vi "Setup Telem APIs.vi"(8 "error in (no error)":errorcluster, 11 "Volatus Core in":refnum<class "Volatus Core.lvclass">) -> (0 "error out":errorcluster, 3 "Volatus Core out":refnum<class "Volatus Core.lvclass">)   [LabVIEW 2020, in "Volatus.lvlib" / "Volatus Core.lvclass"]
uses:
  Volatus Core.lvclass
  C:/dev/lv20CE/relink/lv-volatus/Volatus/Module/Module.lvclass
  Volatus Core.lvclass/Volatus Core.ctl
  Module/Module.lvclass/Module.ctl
  VolatusAPI/VolatusAPI.lvclass/VolatusAPI.ctl
  Module/Module.lvclass
  lv-vecto/Vecto/Vecto/Vecto.lvclass
  VolatusAPI/VolatusAPI.lvclass
  C:/dev/lv20CE/relink/lv-volatus/Volatus/Volatus Core/Volatus Core.lvclass
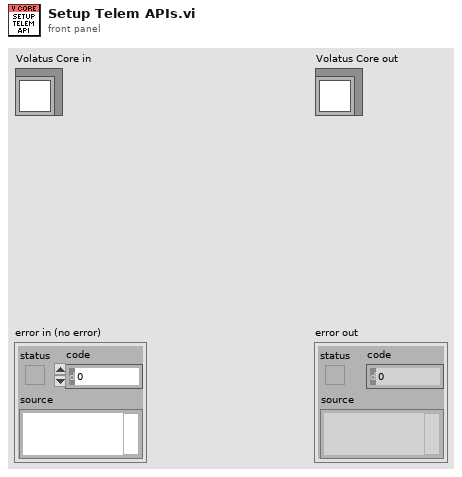
[diagram p1: front panel]
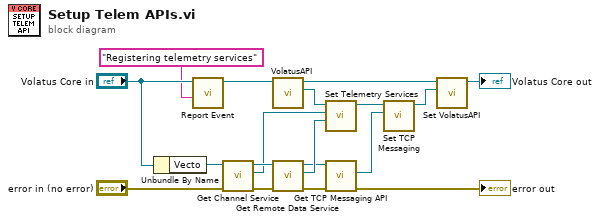
[diagram p0: block diagram]
diagram:
  n1 = Unbundle By Name("Volatus Core in") -> ("Vecto"=w16:refnum<class "Vecto.lvclass">)
  n2 = call "Report Event.vi"("Message"="Registering telemetry services", "Module in"="Volatus Core in") -> ("Module out"=w7:refnum<class "Volatus Core.lvclass">)  [unwired: 8 in, 1 out]
  n3 = call "Get Channel Service.vi"("error in (no error)"="error in (no error)", "Vecto in"=w16) -> ("error out"=w11:errorcluster, "ChannelService"=w13:refnum<class "ChannelService.lvclass">, "Vecto out"=w18:refnum<class "Vecto.lvclass">)  [unwired: 7 in]
  n4 = call "VolatusAPI.vi"("Module in"=w7) -> ("VolatusAPI"=w14:refnum<class "VolatusAPI.lvclass">, "Module out"=w15:refnum<class "Volatus Core.lvclass">)  [unwired: 9 in]
  n5 = call "Get Remote Data Service.vi"("error in (no error)"=w11, "Vecto in"=w18) -> ("error out"=w4:errorcluster, "RemoteDataService"=w12:refnum<class "RemoteDataService.lvclass">, "Vecto out"=w3:refnum<class "Vecto.lvclass">)  [unwired: 7 in]
  n6 = call "Set Telemetry Services.vi"("RemoteDataService"=w12, "ChannelService"=w13, "VolatusAPI in"=w14) -> ("VolatusAPI out"=w8:refnum<class "VolatusAPI.lvclass">)  [unwired: 8 in]
  n7 = call "Get TCP Messaging API.vi"("error in (no error)"=w4, "Vecto in"=w3) -> ("error out"=→"error out":errorcluster, "TCP Messaging API"=w2:refnum<class "TCPMessageAPI.lvclass">)  [unwired: 7 in, 1 out]
  n8 = call "Set TCP Messaging.vi"("Messaging"=w2, "VolatusAPI in"=w8) -> ("VolatusAPI out"=w5:refnum<class "VolatusAPI.lvclass">)  [unwired: 8 in, 1 out]
  n9 = call "Set VolatusAPI.vi"("VolatusAPI"=w5, "Module in"=w15) -> ("Module out"=→"Volatus Core out":refnum<class "Volatus Core.lvclass">)  [unwired: 9 in]
